vi "Autonomous Independent.vi"   [LabVIEW 2018]
doc: "This VI is called when autonomous begins, and will automatically be terminated when autonomous ends. You can carry out timed or sensor driven robot movement independently without needing to return to the caller."
uses:
  <vilib>/Rock Robotics/Network Tables/NT Read String.vi
  <vilib>/Rock Robotics/WPI/Utilities/WPI_GetSetVariantRefNum.vi
  <vilib>/Rock Robotics/Network Tables/NT Write Numeric Array.vi
  Robot Global Data.vi
panel:
  # "Be sure to right-click and choose Data Operations>>Make Current Value default if you want to save the array values with the VI"
types:
  T1 = cluster{"Yaw":dbl, "Roll":dbl, "Pitch":dbl, "Heading":dbl, "Fused Heading":dbl}
  T2 = typedef "WPI_JoystickDevRef.ctl" = cluster{"Device":T3}
  T3 = typedef "WPI_JoystickDeviceEnum.ctl" = enum16{"USB 0", "USB 1", "USB 2", "USB 3", "USB 4", "USB 5"}
  T4 = typedef "WPI_RobotDriveDevRef.ctl" = cluster{"DevStatus":errorcluster, "Motors[]":T5[], "Square Inputs":bool, "Max Output":dbl}
  T5 = typedef "WPI_MotorControlDeviceRef.ctl" = cluster{"DeviceStatus":errorcluster, "Type":T6, "PWM":cluster{"PWM Channel":T7, "DeadBand":T8}, "CAN":cluster{"Device Number":u8, "SetOutput VI Ref":variant, "GetOutput VI Ref":variant, "Enable VI Ref":variant, "Disable VI Ref":variant, "Data":variant}, "Invert":bool, "DIO PWM":cluster{"PWM \"Enable\" Channel":T7, "DIOChannel":T9, "PWM Rate":dbl}}
  T6 = typedef "WPI_MotorControlType.ctl" = enum16{"PWM", "CAN", "DIO PWM"}
  T7 = typedef "FPGA_DIOPWMChannel.ctl" = enum8{"PWM 0", "PWM 1", "PWM 2", "PWM 3", "PWM 4", "PWM 5", "PWM 6", "PWM 7", "PWM 8", "PWM 9", "PWM MXP 0", "PWM MXP 1", "PWM MXP 2", "PWM MXP 3", "PWM MXP 4", "PWM MXP 5", "PWM MXP 6", "PWM MXP 7", "PWM MXP 8", "PWM MXP 9", "Invalid"}
  T8 = typedef "WPI_PWMDeadband.ctl" = cluster{"Name":string, "maxPositivePwm":i32, "minPositivePwm":i32, "centerPwm":i32, "maxNegativePwm":i32, "minNegativePwm":i32, "angularRange":u16}
  T9 = typedef "FPGA_DIOChannel.ctl" = enum8{"DIO 0", "DIO 1", "DIO 2", "DIO 3", "DIO 4", "DIO 5", "DIO 6", "DIO 7", "DIO 8", "DIO 9", "DIO MXP 0", "DIO MXP 1", "DIO MXP 2", "DIO MXP 3", "DIO MXP 4", "DIO MXP 5", "DIO MXP 6", "DIO MXP 7", "DIO MXP 8", "DIO MXP 9", "DIO MXP 10", "DIO MXP 11", "DIO MXP 12", "DIO MXP 13", "DIO MXP 14", "DIO MXP 15", "SPI Port CS1", "SPI Port CS2", "SPI Port CS3", "SPI Port MISO", "SPI Port MOSI", "Invalid"}
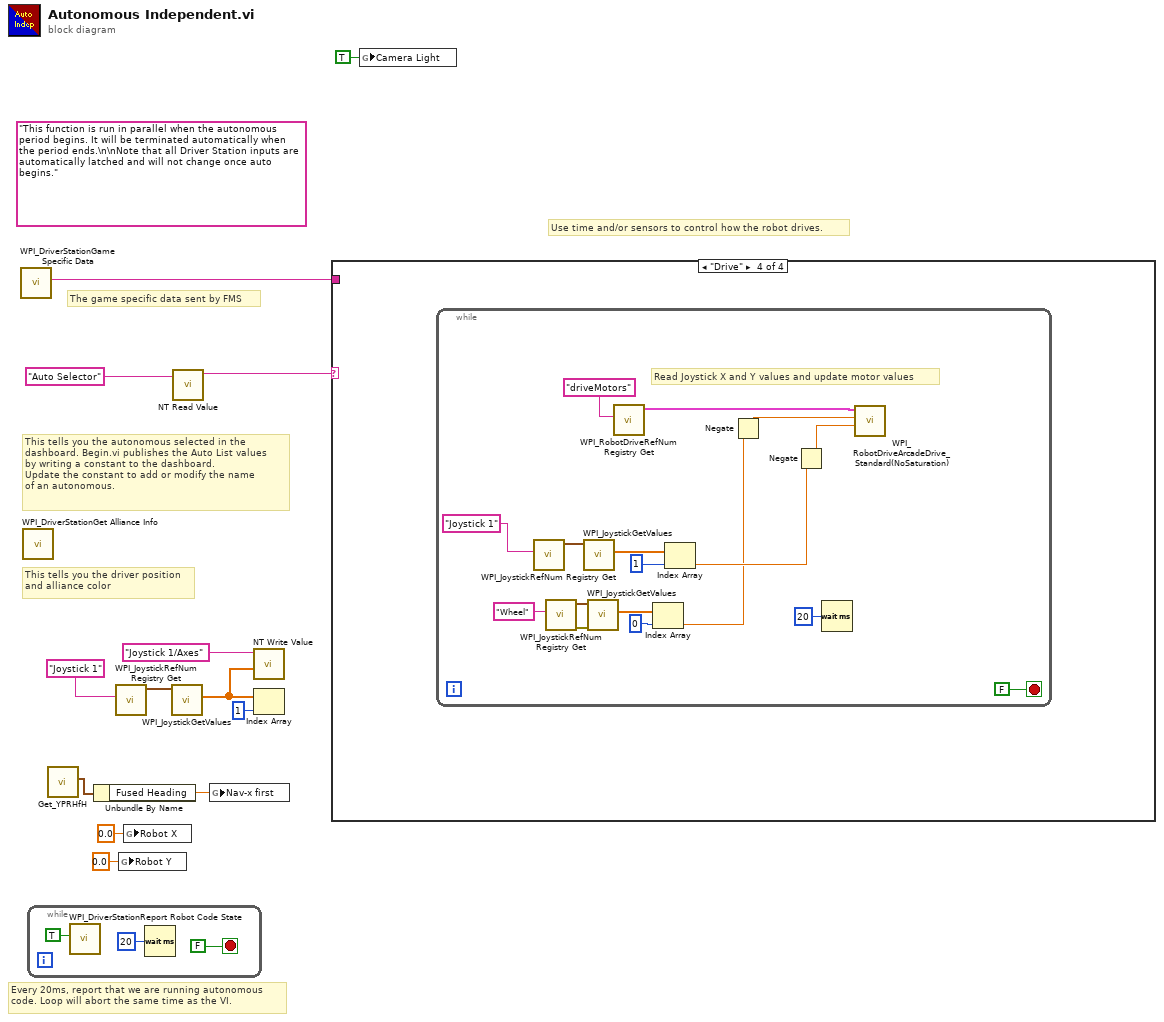
[diagram p0: block diagram]
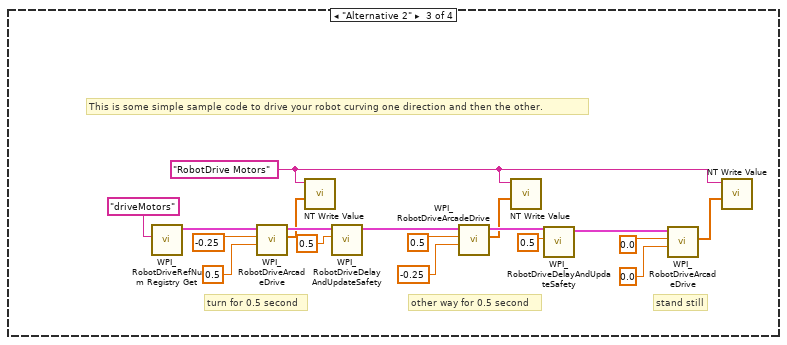
[diagram p4: hidden frame]
diagram:
  (unwired) "This function is run in parallel when the autonomous period begins. It will be terminated automatically when the period ends.\n\nNote that all Driver Station inputs are automatically latched and will not change once auto begins."
  # "The game specific data sent by FMS"
  # "This tells you the autonomous selected in the \ndashboard. Begin.vi publishes the Auto List values\nby writing a constant to the dashboard.\nUpdate the constant to add or modify the name\nof an autonomous."
  # "Every 20ms, report that we are running autonomous\ncode. Loop will abort the same time as the VI."
  # "Use time and/or sensors to control how the robot drives."
  # "This tells you the driver position\nand alliance color"
  n1 = call <vilib>:"WPI_DriverStationGame Specific Data.vi"() -> ("Game Specific Data"=w11:string)  [unwired: 11 in]
  n2 = call <vilib>:"WPI_DriverStationGet Alliance Info.vi"() -> ()  [unwired: 12 out]
  n3 = while {
    stop <- FALSE stop-if-true
    n4 = call <vilib>:"WPI_DriverStationReport Robot Code State.vi"("Autonomous"=TRUE) -> ()  [unwired: 10 in, 1 out]
    n5 = Wait (ms)(milliseconds to wait=u32 20) -> ()  [unwired: 1 out]
  }
  n6 = call <vilib>:"Get_YPRHfH.vi"() -> ("YRPHfH"=w5:T1)  [unwired: 11 in]
  n7 = Unbundle By Name(w5) -> ("Fused Heading"=w4:dbl)
  n8 = call <vilib>:"WPI_JoystickRefNum Registry Get.vi"("refnum name"="Joystick 1") -> ("JoystickDevRef"=w9:T2)  [unwired: 1 in, 9 out]
  n9 = global write "Robot Global Data.vi" "Robot Y"(0.0 ("Robot Y")) -> ()
  n10 = global write "Robot Global Data.vi" "Robot X"(0.0 ("Robot X")) -> ()
  n11 = call <vilib>:"WPI_JoystickGetValues.vi"("JoystickDevRef"=w9) -> ("Axes"=w7:dbl[])  [unwired: 6 in, 4 out]
  n12 = call-poly <vilib>:"NT Read Value.vi"("Name"="Auto Selector") -> ("String"=w12:string)  [unwired: 9 in, 1 out]
  n13 = global write "Robot Global Data.vi" "Nav-x first"(w4) -> ()
  n14 = call-poly <vilib>:"NT Write Value.vi"("Numeric Array"=w7, "Name"="Joystick 1/Axes") -> ()  [unwired: 9 in, 1 out]
  n15 = Index Array(array=w7, index=1) -> ()  [unwired: 1 out]
  n16 = case shown="\"Drive\"" w12 {
    tunnel: w11 -> [_ _ _ _]
    frame Default {
      # "You can put your main auto here, or you can right-click on the case and make any\nother frame be the default case."
      # "This is the frame that will execute if no selection is made, or if it is not recognized"
    }
    frame "Alternative 1" {
    }
    frame "Alternative 2" {
      w18 = "RobotDrive Motors" ("Name")
      # "This is some simple sample code to drive your robot curving one direction and then the other."
      # "stand still"
      # "other way for 0.5 second"
      # "turn for 0.5 second"
      n17 = call <vilib>:"WPI_RobotDriveRefNum Registry Get.vi"("refnum name"="driveMotors") -> ("RobotDriveDevRef"=w34:T4)  [unwired: 1 in, 9 out]
      n18 = call-poly <vilib>:"WPI_RobotDriveArcadeDrive.vi"("Y axis value"=0.5 ("X axis value"), "X axis value"=-0.25, "RobotDriveDevRef"=w34) -> ("Motor Values"=w17:dbl[], "RobotDriveDevRef"=w27:T4)  [unwired: 1 in, 6 out]
      n19 = call-poly <vilib>:"NT Write Value.vi"("Numeric Array"=w17, "Name"=w18) -> ()  [unwired: 9 in, 1 out]
      n20 = call <vilib>:"WPI_RobotDriveDelayAndUpdateSafety.vi"("Delay (s)"=0.5, "RobotDriveDevRef"=w27) -> ("RobotDriveDevRef 2"=w28:T4)  [unwired: 8 in, 1 out]
      n21 = call-poly <vilib>:"WPI_RobotDriveArcadeDrive.vi"("Y axis value"=-0.25 ("X axis value"), "X axis value"=0.5, "RobotDriveDevRef"=w28) -> ("Motor Values"=w19:dbl[], "RobotDriveDevRef"=w29:T4)  [unwired: 1 in, 6 out]
      n22 = call-poly <vilib>:"NT Write Value.vi"("Numeric Array"=w19, "Name"=w18) -> ()  [unwired: 9 in, 1 out]
      n23 = call <vilib>:"WPI_RobotDriveDelayAndUpdateSafety.vi"("Delay (s)"=0.5, "RobotDriveDevRef"=w29) -> ("RobotDriveDevRef 2"=w30:T4)  [unwired: 8 in, 1 out]
      n24 = call-poly <vilib>:"WPI_RobotDriveArcadeDrive.vi"("Y axis value"=0.0 ("X axis value"), "X axis value"=0.0, "RobotDriveDevRef"=w30) -> ("Motor Values"=w20:dbl[])  [unwired: 1 in, 7 out]
      n25 = call-poly <vilib>:"NT Write Value.vi"("Numeric Array"=w20, "Name"=w18) -> ()  [unwired: 9 in, 1 out]
    }
    frame "Drive" {
      n26 = while {
        stop <- FALSE stop-if-true
        # "Read Joystick X and Y values and update motor values"
        n27 = call <vilib>:"WPI_JoystickRefNum Registry Get.vi"("refnum name"="Joystick 1") -> ("JoystickDevRef"=w49:T2)  [unwired: 1 in, 9 out]
        n28 = call <vilib>:"WPI_JoystickRefNum Registry Get.vi"("refnum name"="Wheel") -> ("error out"=w47:errorcluster, "JoystickDevRef"=w46:T2)  [unwired: 9 in]
        n29 = call <vilib>:"WPI_JoystickGetValues.vi"("JoystickDevRef"=w49) -> ("Axes"=w48:dbl[])  [unwired: 6 in, 4 out]
        n30 = call <vilib>:"WPI_JoystickGetValues.vi"("error in (no error)"=w47, "JoystickDevRef"=w46) -> ("Axes"=w45:dbl[])  [unwired: 5 in, 4 out]
        n31 = call <vilib>:"WPI_RobotDriveRefNum Registry Get.vi"("refnum name"="driveMotors") -> ("RobotDriveDevRef"=w50:T4)  [unwired: 1 in, 9 out]
        n32 = Index Array(array=w45, index=0) -> (element=w39:dbl)
        n33 = Index Array(array=w48, index=1) -> (element=w40:dbl)
        n34 = Negate(x=w39) -> (-x=w36:dbl)
        n35 = Negate(x=w40) -> (-x=w35:dbl)
        n36 = Wait (ms)(milliseconds to wait=u32 20) -> ()  [unwired: 1 out]
        n37 = call <vilib>:"WPI_RobotDriveArcadeDrive_Standard(NoSaturation).vi"("Y axis value"=w35, "X axis value"=w36, "RobotDriveDevRef"=w50) -> ()  [unwired: 1 in, 8 out]
      }
    }
  }
  n38 = global write "Robot Global Data.vi" "Camera Light"(TRUE ("Camera Light")) -> ()
